vi "Player.vi"() -> ()   [LabVIEW 2012]
panel:
  in  "Save .wav file":path
  out "Progress":u8(slide) scale=0.0..100.0
  in  "Save output file":bool
  in  "Play after synthesis":bool
  in  "?":bool
  in  "Open .lv file":path
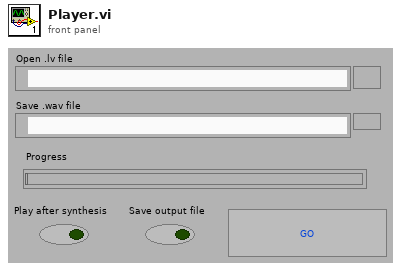
[diagram p1: front panel]
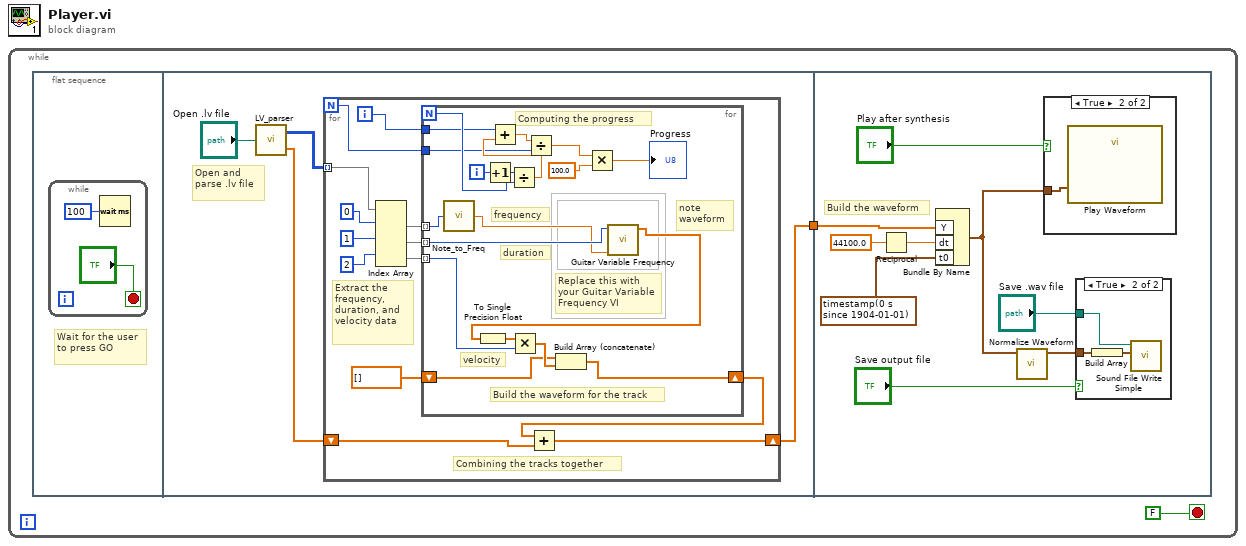
[diagram p0: block diagram]
diagram:
  n1 = while {
    stop <- FALSE stop-if-true
    n2 = flat-sequence {
      tunnel: [w6] -> w1
      tunnel: w1 -> [w47]
      frame #0 {
        # "Wait for the user to press GO"
        n3 = while {
          stop <- "?" stop-if-true
          n4 = Wait (ms)(milliseconds to wait=u32 100) -> ()  [unwired: 1 out]
        }
      }
      frame #1 {
        # "Open and parse .lv file"
        n5 = call "LV_parser.vi"("Open .lv file"="Open .lv file") -> ("Track Array"=w7:i32[][][], "Starting array"=w5:dbl[])
        n6 = for {
          N -> [w14]
          tunnel: w7 -> [w21] mode=indexing
          shift-right: [w10] -> w6
          shift-left: w5 -> [w9]
          i -> [w15]
          # "Combining the tracks together"
          # "Extract the frequency,  duration, and velocity data"
          n7 = Index Array(array=w21, index (row) #1=0 ("index (row)"), index (row) #2=1 ("index (row)"), index (row) #3=2 ("index (row)")) -> (element #1=w18:i32[], element #2=w17:i32[], element #3=w12:i32[])  [unwired: 3 in]
          n8 = for {
            N -> [w40]
            tunnel: w18 -> [w25] mode=indexing
            tunnel: w17 -> [w24] mode=indexing
            shift-right: [w26] -> w11
            shift-left: sgl[] [] -> [w27]
            tunnel: w15 -> [w35]
            tunnel: w14 -> [w33]
            tunnel: w12 -> [w30] mode=indexing
            i -> [w38]
            # "velocity"
            # "Computing the progress"
            # "Build the waveform for the track"
            # "note waveform"
            # "duration"
            # "frequency"
            # "Replace this with your Guitar Variable Frequency VI"
            n9 = call "Note_to_Freq.vi"("note"=w25) -> ("frequency"=w23:sgl)
            n10 = Increment(x=w38) -> (x+1=w39:i32)
            n11 = Divide(x=w39, y=w40) -> (x/y=w34:dbl)
            n12 = Add(x=w35, y=w34) -> (x+y=w36:dbl)
            n13 = Divide(x=w36, y=w33) -> (x/y=w32:dbl)
            n14 = Multiply(x=w32, y=100.0 ("x")) -> (x*y=→"Progress":dbl)
            n15 = call "Guitar Variable Frequency.vi"("Frequency"=w23, "Samples"=w24) -> ("Array"=w22:dbl[])  [unwired: 9 in]
            n16 = To Single Precision Float(number=w22) -> (single precision float=w28:sgl[])
            n17 = Multiply(x=w28, y=w30) -> (x*y=w29:sgl[])
            n18 = Build Array (concatenate)(w27, w29) -> (w26:sgl[])
          }
          n19 = Add(x=w11, y=w9) -> (x+y=w10:dbl[])
        }
      }
      frame #2 {
        # "Build the waveform"
        n20 = Reciprocal(x=44100.0) -> (1/x=w46:dbl)
        n21 = Bundle By Name("Y"=w47, "dt"=w46, "t0"=timestamp(0 s since 1904-01-01)) -> (w41:waveform(dbl))  [unwired: 1 in]
        n22 = call <vilib>:"Normalize Waveform.vi"("waveform in"=w41) -> ("normalized waveform"=w42:waveform(dbl))  [unwired: 7 in, 3 out]
        n23 = case shown="True" "Play after synthesis" {
          tunnel: w41 -> [_ w53]
          frame False {
          }
          frame True {
            n24 = call "Play Waveform"("Data"=w53) -> ()  [unwired: 18 in, 1 out]
          }
        }
        n25 = case shown="True" "Save output file" {
          tunnel: w42 -> [_ w52]
          tunnel: "Save .wav file" -> [_ w50]
          frame False {
          }
          frame True {
            n26 = Build Array(w52) -> (w51:waveform(dbl)[])
            n27 = call <vilib>:"Sound File Write Simple.vi"("data"=w51, "path"=w50) -> ()  [unwired: 8 in, 2 out]
          }
        }
      }
    }
  }
